vi "REmoveSpacesInRow.vi"(11 "Array":string[](array[string])) -> (3 "outArray":string[](array[string]))   [LabVIEW 2023]
uses:
  <vilib>/Utility/error.llb/Trim Whitespace One-Sided.vi
panel:
  in  "String":string
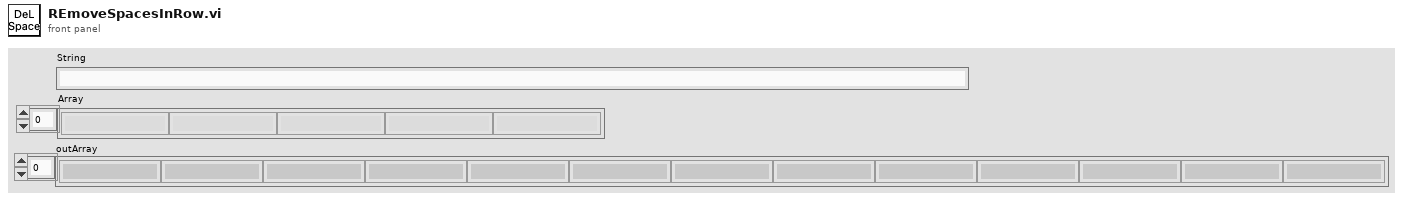
[diagram p1: front panel]
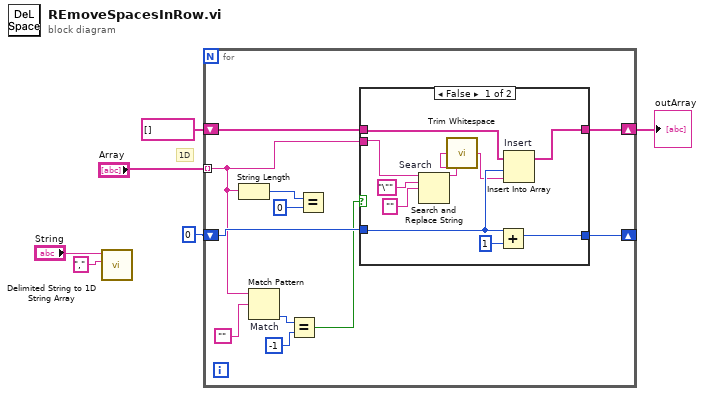
[diagram p0: block diagram]
diagram:
  # "1D"
  n1 = call <vilib>:"Delimited String to 1D String Array.vi"("delimiter"="," ("delimiter (Tab)"), "delimited string"="String") -> ()  [unwired: 9 in, 1 out]
  n2 = for {
    tunnel: "Array" -> [w12] mode=indexing
    shift-right: [w7] -> w2
    shift-left: string[] [] -> [w17]
    shift-right: [w16] -> _
    shift-left: 0 ("y") -> [w15]
    n3 = String Length(string=w12) -> (length=w13:i32)
    n4 = Match Pattern "Match"(string=w12, regular expression="") -> (offset past match=w11:i32)  [unwired: 1 in, 3 out]
    n5 = Equal?(x=w11, y=-1) -> (x = y?=w9:bool)
    n6 = Equal?(x=w13, y=0) -> ()  [unwired: 1 out]
    n7 = case shown="False" w9 {
      tunnel: w12 -> [w22 _]
      tunnel: [w27 w28] -> w7
      tunnel: w17 -> [w26 w28]
      tunnel: [w23 w29] -> w16
      tunnel: w15 -> [w24 w29]
      frame False {
        n8 = Search and Replace String "Search"(input string=w22, search string="\"", replace string="" ("replace string (\"\")")) -> (result string=w19:string)  [unwired: 5 in, 3 out]
        n9 = call <vilib>:"Trim Whitespace.vi"("string"=w19) -> ("trimmed string"=w18:string)  [unwired: 1 in]
        n10 = Add(x=w24, y=1) -> (x+y=w23:i32)
        n11 = Insert Into Array "Insert"(array=w26, index=w24, new element=w18) -> (w27:string[])
      }
      frame True {
      }
    }
  }
  "outArray" <- w2
